vi "ActivateStepDirectionMode.vi"(4 "error in (no error)":errorcluster, 6 "step direction parameter":T1, 7 "axis in":cluster{"keyHandle":u32, "nodeId":u16}={"keyHandle"=0, "nodeId"=1}) -> (0 "error out":errorcluster, 3 "axis out":cluster{"keyHandle":u32, "nodeId":u16}={"keyHandle"=0, "nodeId"=1})   [LabVIEW 2017, in "maxonEPOS.lvlib"]
doc: "<B>ActivateStepDirectionMode</B> changes the operational mode to step direction mode (SDM)."
uses:
  Examples/maxonEPOS.lvlib
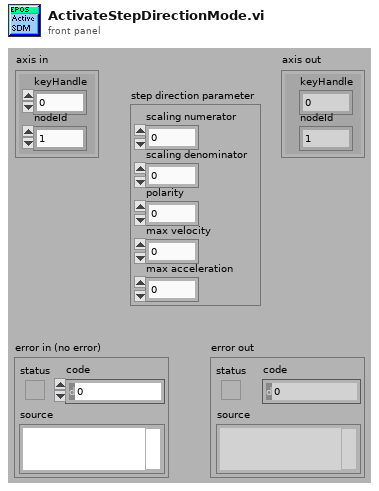
[diagram p1: front panel]
types:
  T1 = cluster{"scaling numerator":u16, "scaling denominator":u16, "polarity":u8, "max velocity":u32, "max acceleration":u32}
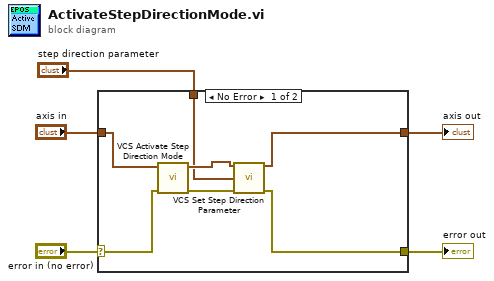
[diagram p0: block diagram]
diagram:
  n1 = case shown="No Error" "error in (no error)" {
    selector: "error in (no error)" -> [w7 w14]
    tunnel: [w9 w14] -> w4
    tunnel: [w10 w13] -> w3
    tunnel: "axis in" -> [w12 w13]
    tunnel: "step direction parameter" -> [w6 _]
    frame No Error {
      n2 = call "VCS Activate Step Direction Mode.vi"("error in (no error)"=w7, "axis in"=w12) -> ("error out"=w8:errorcluster, "axis out"=w11:cluster{"keyHandle":u32, "nodeId":u16})  [unwired: 8 in]
      n3 = call "VCS Set Step Direction Parameter.vi"("axis in"=w11, "step direction parameter"=w6, "error in (no error)"=w8) -> ("axis out"=w10:cluster{"keyHandle":u32, "nodeId":u16}, "error out"=w9:errorcluster)  [unwired: 11 in]
    }
    frame Error {
    }
  }
  "error out" <- w4
  "axis out" <- w3
